vi "TIFF Append New IFD.vi"(9 "Last Reference Offset":u32, 10 "refnum in":refnum<file>, 11 "IFD in":refnum<class "IFD.lvclass">) -> (1 "Reference Offset":u32, 2 "refnum out":refnum<file>)   [LabVIEW 2016]
uses:
  Class/IFD/IFD.lvclass
  Class/IFD/IFD.lvclass/IFD.ctl
  Class/Tag/IFD_Tag.lvclass/IFD_Tag.ctl
  Class/IFD/IFD Tag Total Size.vi
  Class/Tag/Tag ID.vi
  Class/Tag/Tag Data.vi
  Class/Tag/Tag Change Value.vi
  Class/IFD/Image Data/IFD U16 Image out.vi
  Class/IFD/Image Data/IFD RGB Image out.vi
  Class/IFD/Image Data/IFD SGL Image out.vi
  Class/Tag/Tag Size.vi
  Class/Tag/Tag Write to File.vi
  Class/IFD/Write All Pending Data.vi
  Class/Tag/IFD_Tag.lvclass
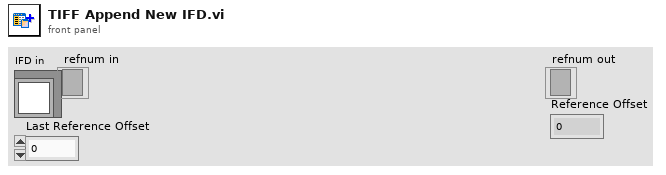
[diagram p1: front panel]
types:
  T1 = enum16{"big-endian, network order", "native, host order", "little-endian"}
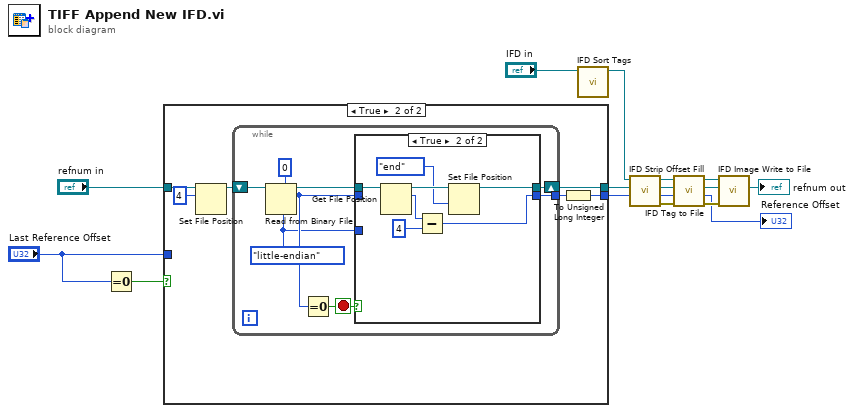
[diagram p0: block diagram]
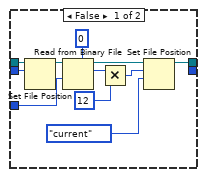
[diagram p3: hidden frame]
diagram:
  n1 = Equal To 0?(x="Last Reference Offset") -> (x = 0?=w15:bool)
  n2 = case shown="True" w15 {
    tunnel: "Last Reference Offset" -> [w17 _]
    tunnel: [w17 w18] -> w13
    tunnel: "refnum in" -> [w16 w23]
    tunnel: [w16 w20] -> w10
    frame False {
    }
    frame True {
      n3 = Set File Position(offset (in bytes) (0)=i64 4, refnum=w23) -> (refnum out=w21:refnum<file>)  [unwired: 2 in, 1 out]
      n4 = while {
        shift-right: [w27] -> w20
        shift-left: w21 -> [w31]
        tunnel: [w26] -> w19
        stop <- w29 stop-if-true
        w24 = T1."little-endian" ("byte order (0:big-endian, network order)")
        n5 = Read from Binary File(5:u32 0, 9:w24, 11:w31) -> (2:w25:u32, 3:w28:refnum<file>)  [unwired: 3 in, 2 out]
        n6 = Equal To 0?(x=w25) -> (x = 0?=w29:bool)
        n7 = case shown="True" w29 {
          tunnel: w28 -> [w42 w49]
          tunnel: [w33 w44] -> w27
          tunnel: [_ w45] -> w26
          tunnel: w25 -> [w41 _]
          tunnel: w24 -> [w32 _]
          frame False {
            n8 = Set File Position(offset (in bytes) (0)=w41, refnum=w42) -> (refnum out=w40:refnum<file>)  [unwired: 2 in, 1 out]
            n9 = Read from Binary File(5:u16 0, 9:w32, 11:w40) -> (2:w36:u16, 3:w38:refnum<file>)  [unwired: 3 in, 2 out]
            n10 = Multiply(x=w36, y=i64 12) -> (x*y=w34:i64)
            n11 = Set File Position(offset (in bytes) (0)=w34, refnum=w38, from (0:start)=enum16{"start", "end", "current"}."current") -> (refnum out=w33:refnum<file>)  [unwired: 1 in, 1 out]
          }
          frame True {
            n12 = Get File Position(7:w49) -> (2:w47:i64, 3:w48:refnum<file>)  [unwired: 1 in, 1 out]
            n13 = Subtract(x=w47, y=i64 4) -> (x-y=w45:i64)
            n14 = Set File Position(refnum=w48, from (0:start)=enum16{"start", "end", "current"}."end") -> (refnum out=w44:refnum<file>)  [unwired: 2 in, 1 out]
          }
        }
      }
      n15 = To Unsigned Long Integer(number=w19) -> (unsigned 32bit integer=w18:u32)
    }
  }
  n16 = call "IFD Sort Tags.vi"("IFD in"="IFD in") -> ("IFD out"=w9:refnum<class "IFD.lvclass">)  [unwired: 9 in, 1 out]
  n17 = call "IFD Strip Offset Fill.vi"("refnum"=w10, "IFD in"=w9) -> ("error out"=w4:errorcluster, "refnum out"=w7:refnum<file>, "IFD out"=w8:refnum<class "IFD.lvclass">)  [unwired: 7 in]
  n18 = call "IFD Tag to File.vi"("error in (no error)"=w4, "Last Reference Offset"=w13, "refnum in"=w7, "IFD in"=w8) -> ("error out"=w3:errorcluster, "Reference Offset"=→"Reference Offset":u32, "refnum out"=w5:refnum<file>, "IFD out"=w6:refnum<class "IFD.lvclass">)  [unwired: 4 in]
  n19 = call "IFD Image Write to File.vi"("error in (no error)"=w3, "refnum in"=w5, "IFD in"=w6) -> ("refnum out"=→"refnum out":refnum<file>)  [unwired: 7 in, 1 out]
